vi "Convert_Decimal_Degrees_to DMS.vi"(4 "Decimal Degrees":sgl) -> (0 "Seconds":i16, 1 "Minutes":i16, 2 "Degrees":i16)   [LabVIEW 2015]
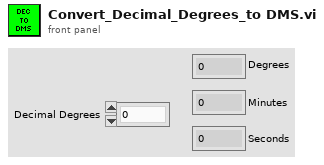
[diagram p1: front panel]
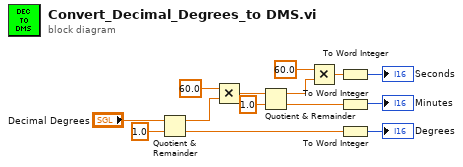
[diagram p0: block diagram]
diagram:
  n1 = Quotient & Remainder(x="Decimal Degrees", y=sgl 1.0) -> (x-y*floor(x/y)=w7:sgl, floor(x/y)=w11:sgl)
  n2 = Multiply(x=sgl 60.0, y=w7) -> (x*y=w9:sgl)
  n3 = Quotient & Remainder(x=w9, y=sgl 1.0) -> (x-y*floor(x/y)=w2:sgl, floor(x/y)=w6:sgl)
  n4 = Multiply(x=sgl 60.0, y=w2) -> (x*y=w1:sgl)
  n5 = To Word Integer(number=w1) -> (16bit integer=→"Seconds":i16)
  n6 = To Word Integer(number=w6) -> (16bit integer=→"Minutes":i16)
  n7 = To Word Integer(number=w11) -> (16bit integer=→"Degrees":i16)
